vi "Get Wii State.vi"(8 "error in (no error)":errorcluster, 9 "Wiimote Player #":i32, 11 "LV Wiimote Interface in":T1) -> (0 "error out":errorcluster, 2 "WiimoteState":refnum<k24>, 3 "LV Wiimote Interface out":T1)   [LabVIEW 2012, in "LV Wiimote Interface.lvclass"]
uses:
  LV Wiimote Interface.lvclass
  C:/Program Files/National Instruments/LabVIEW 2012/vi.lib/LabVIEW Hacker/WiiMote/Dependencies/WiimoteLib.dll
  Program Files/National Instruments/LabVIEW 2012/vi.lib/LabVIEW Hacker/WiiMote/Dependencies/WiimoteLib.dll
  Controls/LV Wiimote Interface.ctl
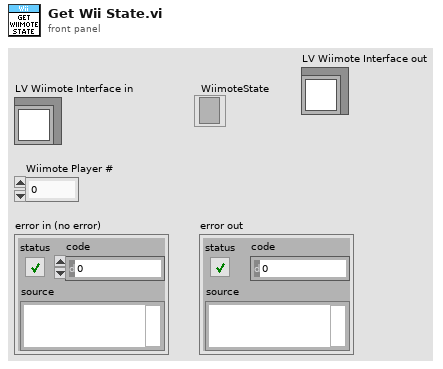
[diagram p1: front panel]
types:
  T1 = typedef "LV Wiimote Interface.ctl" = refnum<class "LV Wiimote Interface.lvclass">
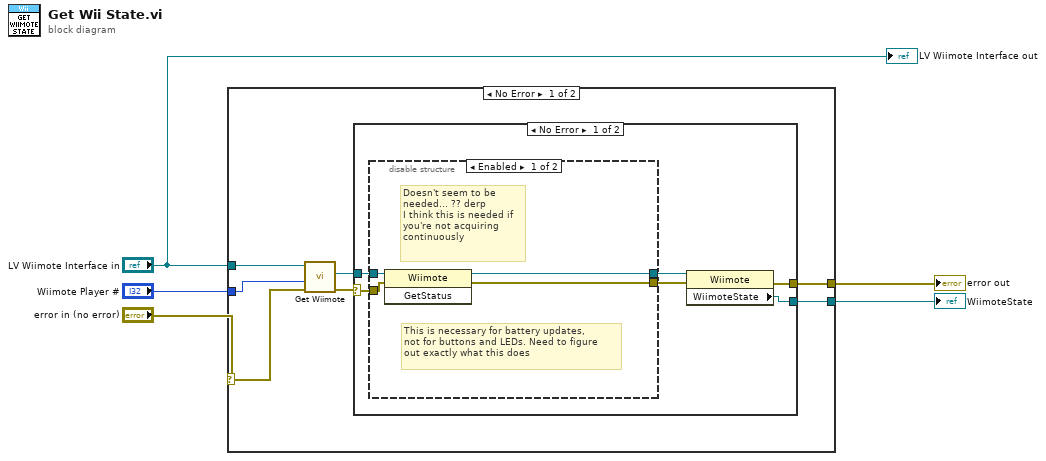
[diagram p0: block diagram]
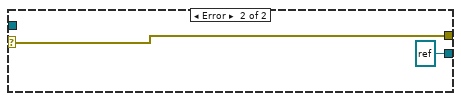
[diagram p3: hidden frame]
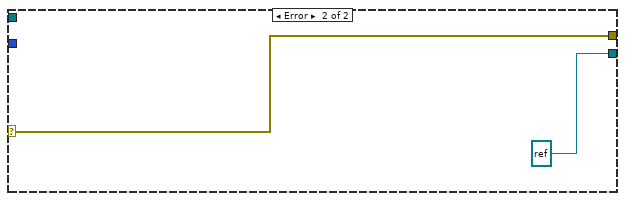
[diagram p4: hidden frame]
diagram:
  n1 = case shown="No Error" "error in (no error)" {
    selector: "error in (no error)" -> [w9 w28]
    tunnel: "Wiimote Player #" -> [w6 _]
    tunnel: [w12 w28] -> w4
    tunnel: "LV Wiimote Interface in" -> [w11 _]
    tunnel: [w8 refnum<k24> refnum ("WiimoteState")] -> w1
    frame No Error {
      n2 = call "Get Wiimote.vi"("error in (no error)"=w9, "Wiimote Player #"=w6, "LV Wiimote Interface in"=w11) -> ("error out"=w7:errorcluster, "Wiimote"=w10:refnum<k24>)  [unwired: 6 in, 1 out]
      n3 = case shown="No Error" w7 {
        selector: w7 -> [w13 w26]
        tunnel: [w16 w26] -> w12
        tunnel: w10 -> [w15 _]
        tunnel: [w14 refnum<k24> refnum ("WiimoteState")] -> w8
        frame No Error {
          n4 = disable-structure shown="Enabled" {
            disable-tunnel: w15 -> [w22 w23]
            disable-tunnel: [w21 w23] -> w17
            disable-tunnel: [w20 w24] -> w18
            disable-tunnel: w13 -> [w19 w24]
            frame Enabled {
              # "This is necessary for battery updates, \nnot for buttons and LEDs. Need to figure \nout exactly what this does"
              # "Doesn't seem to be \nneeded... ?? derp\nI think this is needed if \nyou're not acquiring \ncontinuously"
              n5 = invoke class="Wiimote" method="GetStatus"(reference=w22, error in=w19) -> (reference out=w21:refnum<k24>, error out=w20:errorcluster)  [unwired: 1 in, 1 out]
            }
            frame Disabled {
            }
          }
          n6 = property class="Wiimote"(reference=w17, error in=w18) -> (error out=w16:errorcluster, "WiimoteState"=w14:refnum<k24>)  [unwired: 1 out]
        }
        frame Error {
        }
      }
    }
    frame Error {
    }
  }
  "error out" <- w4
  "WiimoteState" <- w1
  "LV Wiimote Interface out" <- "LV Wiimote Interface in"
